vi "Propagate.vi"(11 "AER in":refnum<class "AER.lvclass">) -> (3 "AER out":refnum<class "AER.lvclass">)   [LabVIEW 2013, in "AER.lvclass"]
doc: "This VI calculates the currents of each neuron using the AER inverse implementation. MFs are bypassed because there are propagated in a separate Vi"
uses:
  AER.lvclass
  Controls/Type of Neuron.ctl
  AER.lvclass/AER.ctl
panel:
  out "Firing rates":dbl[](graph)
  out "From":i32
  out "To":i32
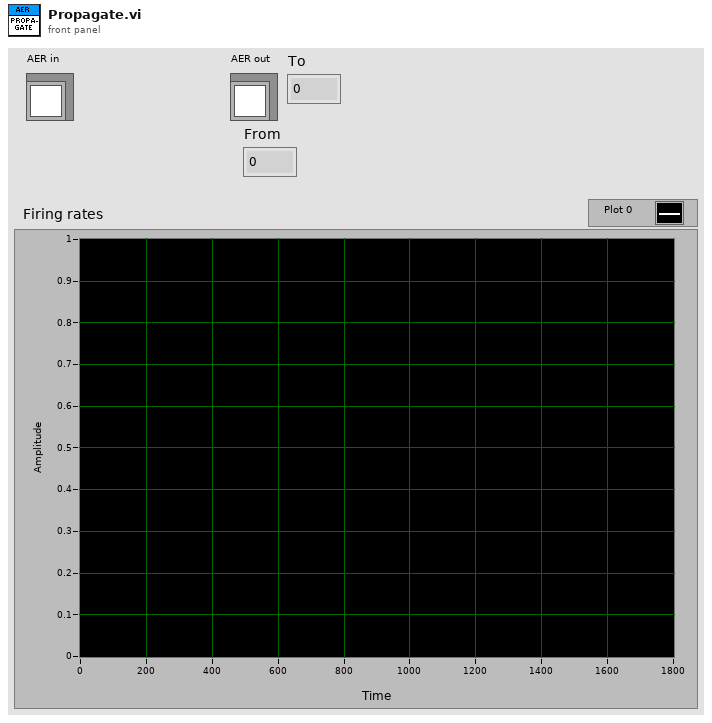
[diagram p1: front panel]
types:
  T1 = typedef "Type of Neuron.ctl" = enum16{"MF", "BA", "GO", "GC", "PC", "LU", "Glia (Dummy)"}
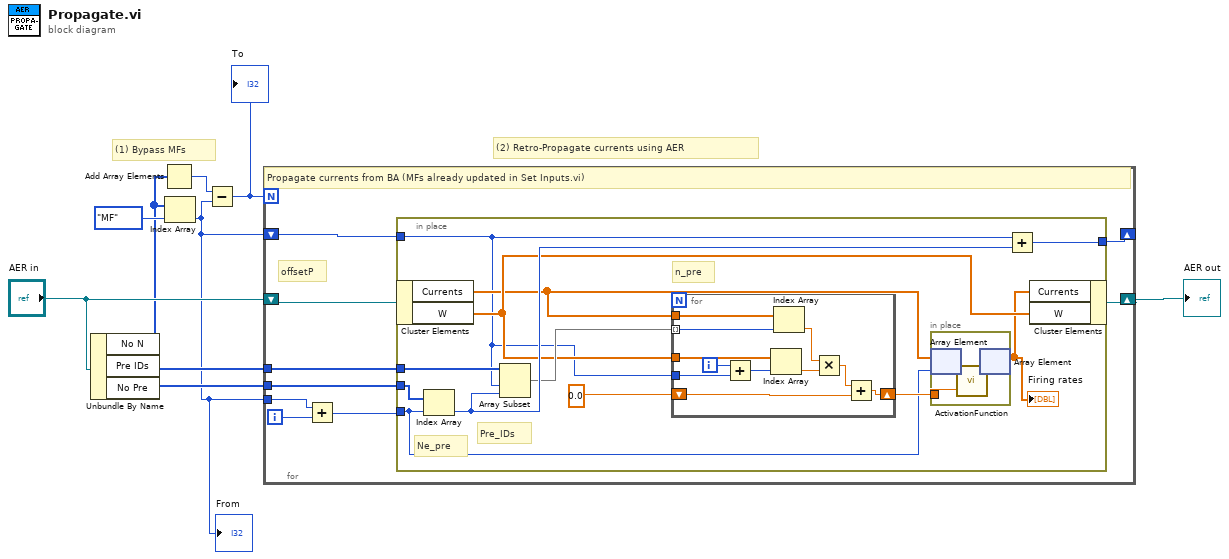
[diagram p0: block diagram]
diagram:
  # "(2) Retro-Propagate currents using AER"
  # "(1) Bypass MFs"
  n1 = Unbundle By Name("AER in") -> ("No N"=w5:i32[], "Pre IDs"=w9:i32[], "No Pre"=w8:i32[])
  n2 = Add Array Elements(numeric array=w5) -> (sum=w4:i32)
  n3 = Index Array(array=w5, index=Type_of_Neuron."MF" ("Type of Neuron")) -> (element=w1:i32)
  "From" <- w1
  n4 = Subtract(x=w4, y=w1) -> (x-y=w3:i32)
  "To" <- w3
  n5 = for {
    N: w3 -> [_]
    tunnel: w8 -> [w18]
    shift-right: [w13] -> w2
    shift-left: "AER in" -> [w14]
    shift-right: [w17] -> _
    shift-left: w1 -> [w15]
    tunnel: w9 -> [w16]
    tunnel: w1 -> [w10]
    i -> [w12]
    # "offsetP"
    # "Propagate currents from BA (MFs already updated in Set Inputs.vi)"
    n6 = Add(x=w10, y=w12) -> (x+y=w11:i32)
    n7 = in-place {
      in-place-border: w18 -> [w29]
      in-place-border: [w28] -> w17
      in-place-border: w16 -> [w27]
      in-place-border: w15 -> [w20]
      in-place-border: w11 -> [w23]
      # "n_pre"
      # "Pre_IDs"
      # "Ne_pre"
      n8 = in-place-cluster #1(w14) -> ("Currents"=w21:dbl[], "W"=w22:dbl[])
      n9 = Index Array(array=w29, index=w23) -> (element=w25:i32)
      n10 = Array Subset(array=w27, index=w20, length=w25) -> (w24:i32[])
      n11 = for {
        shift-right: [w39] -> w30
        shift-left: 0.0 ("N") -> [w41]
        tunnel: w22 -> [w43]
        tunnel: w20 -> [w40]
        tunnel: w24 -> [w33] mode=indexing
        tunnel: w21 -> [w34]
        i -> [w35]
        n12 = Add(x=w35, y=w40) -> (x+y=w38:i32)
        n13 = Index Array(array=w43, index=w38) -> (element=w42:dbl)
        n14 = Index Array(array=w34, index=w33) -> (element=w36:dbl)
        n15 = Multiply(x=w36, y=w42) -> (x*y=w37:dbl)
        n16 = Add(x=w37, y=w41) -> (x+y=w39:dbl)
      }
      n17 = in-place {
        in-place-border: w30 -> [w32]
        n18 = in-place-array #2(w21, w23) -> ()  [unwired: 1 out]
        n19 = call "ActivationFunction.vi"("x"=w32) -> ("y"=w31:dbl)  [unwired: 2 in]
        n20 = in-place-array #2(w31) -> (w19:dbl[])  [unwired: 1 out]
      }
      "Firing rates" <- w19
      n21 = Add(x=w20, y=w25) -> (x+y=w28:i32)
      n22 = in-place-cluster #1("Currents"=w19, "W"=w22) -> (w13:refnum<class "AER.lvclass">)
    }
  }
  "AER out" <- w2
